vi "Text_Select Valid Font.vi"(8 "Error":errorcluster, 11 "Font":string) -> (0 "Error Out":errorcluster, 3 "Valid Font Name Out":string, 5 "Font List Out":string[](array[string]))   [LabVIEW 2021]
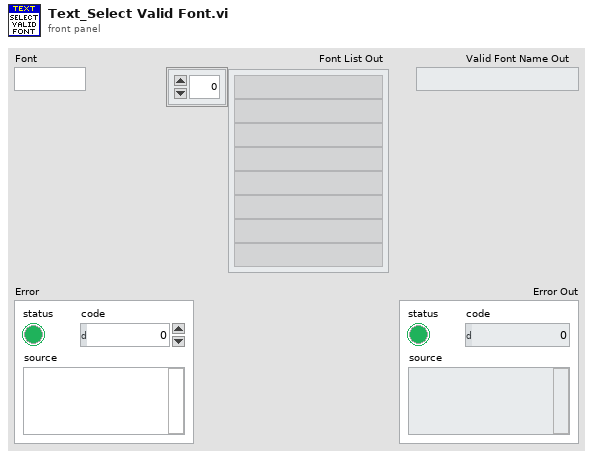
[diagram p1: front panel]
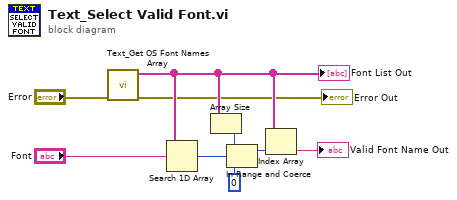
[diagram p0: block diagram]
diagram:
  n1 = call "Text_Get OS Font Names Array.vi"("Error"="Error") -> ("Error Out"=→"Error Out":errorcluster, "Font Names Array Out"=w2:string[])  [unwired: 9 in]
  "Font List Out" <- w2
  n2 = Search 1D Array(1D array=w2, element="Font") -> (index of element=w6:i32)  [unwired: 1 out]
  n3 = Array Size(array=w2) -> (size(s)=w9:i32)
  n4 = In Range and Coerce(upper limit=w9, x=w6, lower limit=0 ("x")) -> (coerced(x)=w8:i32)  [unwired: 1 out]
  n5 = Index Array(array=w2, index=w8) -> (element=→"Valid Font Name Out":string)
